vi "DriveForDistance.vi"(8 "error in (no error)":errorcluster, 9 "RobotDriveRef":T1={"RobotDriveDevRef"={"DevStatus"={"status"=FALSE, "code"=0, "source"=""}, "Motors[]"=[], "Square Inputs"=FALSE, "Max Output"=0.0}, "Control Mode"=enum."Percent VBus", "Motor Settings"={"Wheel Radius"=0.0, "Encoder Ticks Per Rev"=0.0, "Gear Ratio"=0.0, "ClimbRev"=0.0}, "Default Control Mode"=enum."Unchanged / Invalid"}, 10 "SubSystem Data":T10, 11 "Command Loop Data":cluster{"Start Time (ms)":u32, "Iterations":i32}) -> (0 "error out":errorcluster, 1 "RobotDriveRef Out":T1={"RobotDriveDevRef"={"DevStatus"={"status"=FALSE, "code"=0, "source"=""}, "Motors[]"=[], "Square Inputs"=FALSE, "Max Output"=0.0}, "Control Mode"=enum."Percent VBus", "Motor Settings"={"Wheel Radius"=0.0, "Encoder Ticks Per Rev"=0.0, "Gear Ratio"=0.0, "ClimbRev"=0.0}, "Default Control Mode"=enum."Unchanged / Invalid"}, 2 "Wait Time":dbl, 3 "Finished":bool, 5 "Left Setpoint":dbl)   [LabVIEW 2015]
uses:
  Drive Setpoints.ctl
  Drive Operations.ctl
  Advanced Drive VIs/RobotDrive Type Def.ctl
  <vilib>/Rock Robotics/WPI/MotorControl/WPI_MotorControlDeviceRef.ctl
  <vilib>/Rock Robotics/WPI/MotorControl/WPI_MotorControlType.ctl
  <vilib>/Rock Robotics/SystemInterfaces/DIO/FPGA_DIOPWMChannel.ctl
  <vilib>/Rock Robotics/WPI/PWM/WPI_PWMDeadband.ctl
  <vilib>/Rock Robotics/WPI/CAN/Jaguar/SubVIs/WPI_CANJaguar_ControlMode.ctl
  <vilib>/Rock Robotics/WPI/CAN/TalonSRX/WPI_CANTalonSRX_APIControlMode.ctl
  Advanced Drive VIs/Drive Motor Settings.ctl
panel:
  out "x*y":dbl
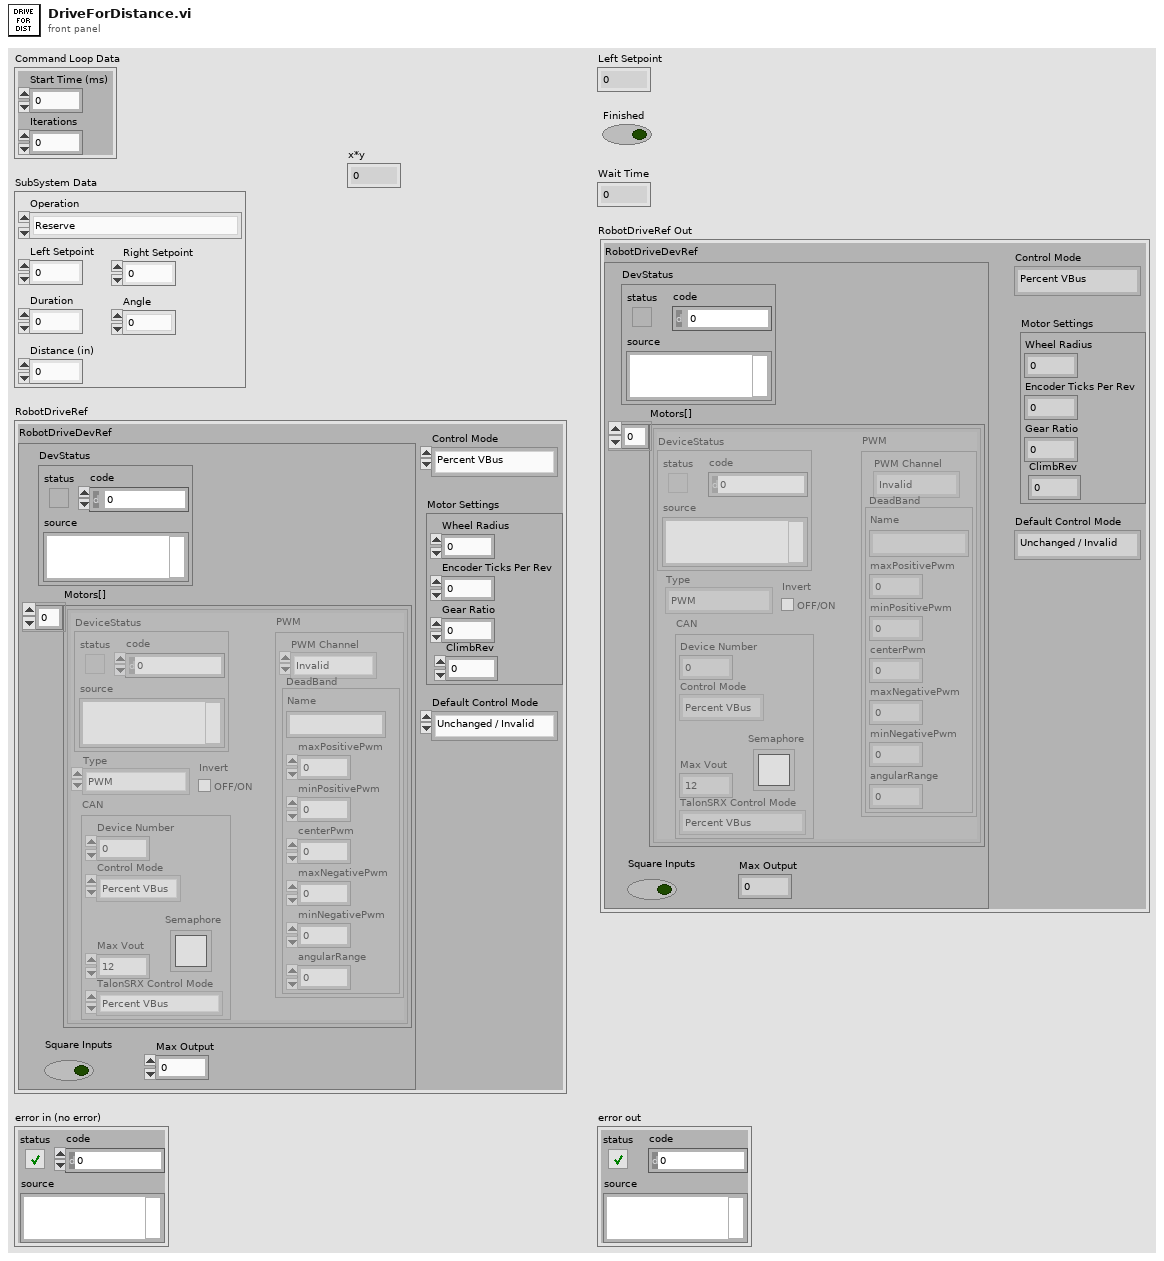
[diagram p1: front panel]
types:
  T1 = typedef "RobotDrive Type Def.ctl" = cluster{"RobotDriveDevRef":cluster{"DevStatus":errorcluster, "Motors[]":T2[], "Square Inputs":bool, "Max Output":dbl}, "Control Mode":T8, "Motor Settings":T9, "Default Control Mode":T8}
  T2 = typedef "WPI_MotorControlDeviceRef.ctl" = cluster{"DeviceStatus":errorcluster, "Type":T3, "PWM":cluster{"PWM Channel":T4, "DeadBand":T5}, "CAN":cluster{"Device Number":u8, "Control Mode":T6, "Semaphore":T7, "Max Vout":dbl, "TalonSRX Control Mode":T8}, "Invert":bool}
  T3 = typedef "WPI_MotorControlType.ctl" = enum16{"PWM", "CAN", "CANTalonSRX"}
  T4 = typedef "FPGA_DIOPWMChannel.ctl" = enum8{"PWM 0", "PWM 1", "PWM 2", "PWM 3", "PWM 4", "PWM 5", "PWM 6", "PWM 7", "PWM 8", "PWM 9", "PWM MXP 0", "PWM MXP 1", "PWM MXP 2", "PWM MXP 3", "PWM MXP 4", "PWM MXP 5", "PWM MXP 6", "PWM MXP 7", "PWM MXP 8", "PWM MXP 9", "Invalid"}
  T5 = typedef "WPI_PWMDeadband.ctl" = cluster{"Name":string, "maxPositivePwm":i32, "minPositivePwm":i32, "centerPwm":i32, "maxNegativePwm":i32, "minNegativePwm":i32, "angularRange":u16}
  T6 = typedef "WPI_CANJaguar_ControlMode.ctl" = enum8{"Percent VBus", "Current", "Speed", "Position", "Voltage"}
  T7 = typedef "Semaphore RefNum" = refnum<k1>
  T8 = typedef "WPI_CANTalonSRX_APIControlMode.ctl" = enum8{"Percent VBus", "Speed", "Position", "Slave", "Unchanged / Invalid", "Voltage Compensation", "Current", "Motion Profile"}
  T9 = typedef "Drive Motor Settings.ctl" = cluster{"Wheel Radius":dbl, "Encoder Ticks Per Rev":dbl, "Gear Ratio":dbl, "ClimbRev":dbl}
  T10 = typedef "Drive Setpoints.ctl" = cluster{"Operation":T11, "Left Setpoint":dbl, "Right Setpoint":dbl, "Duration":dbl, "Angle":dbl, "Distance (in)":dbl}
  T11 = typedef "Drive Operations.ctl" = enum16{"Reserve", "Read Current", "Immediate", "Drive for Time", "Drive for Distance", "Turn Degrees"}
  T12 = typedef "WPI_CANTalonSRX_GlobalStatus.ctl" = cluster{"Applied Throttle":dbl, "Module Enabled":bool, "CAN Error":errorcluster, "Closed Loop Error":dbl, "Forward Limit Switch Closed":bool, "Reverse Limit Switch Closed":bool, "Sensor Position":dbl, "Sensor Velocity":dbl, "Current":dbl, "Sticky Fault - Over Temp":bool, "Sticky Fault - Under Voltage":bool, "Sticky Fault - Forward Limit":bool, "Sticky Fault - Reverse Limit":bool, "Sticky Fault - Forward Soft Limit":bool, "Sticky Fault - Reverse Soft Limit":bool, "Brake is Enabled":bool, "Encoder Position":dbl, "Encoder Velocity":dbl, "Encoder Index Count":dbl, "Encoder A Pin State":bool, "Encoder B Pin State":bool, "Encoder Index Pin State":bool, "Analog In":dbl, "Analog In Velocity":dbl, "Temperature (C)":dbl, "Battery Voltage":dbl, "Control 5 Is Supported":bool, "Current Profile Slot Select":dbl, "Pos Div 8":bool, "Vel Div 4":bool, "Pulse Width Position":i32, "Pulse Width Velocity":i32, "Pulse Width Rise To Rise (us)":i32, "Pulse Width Rise To Fall (us)":i32, "Mot Prof Active Is Under Run":bool, "Mot Prof Active Has Under Run":bool, "Mot Prof Active Is Last":bool, "Mot Prof Active Velocity Only":bool, "Mot Prof Active Is Valid":bool, "Mot Prof Buffer Is Full":bool, "Mot Prof Active Profile Slot Select":i32, "Mot Prof NextID":i32, "Mot Prof Count":i32, "Mot Prof Active Velocity":dbl, "Mot Prof Active Position":dbl, "Mot Prof Output Enable":i32}
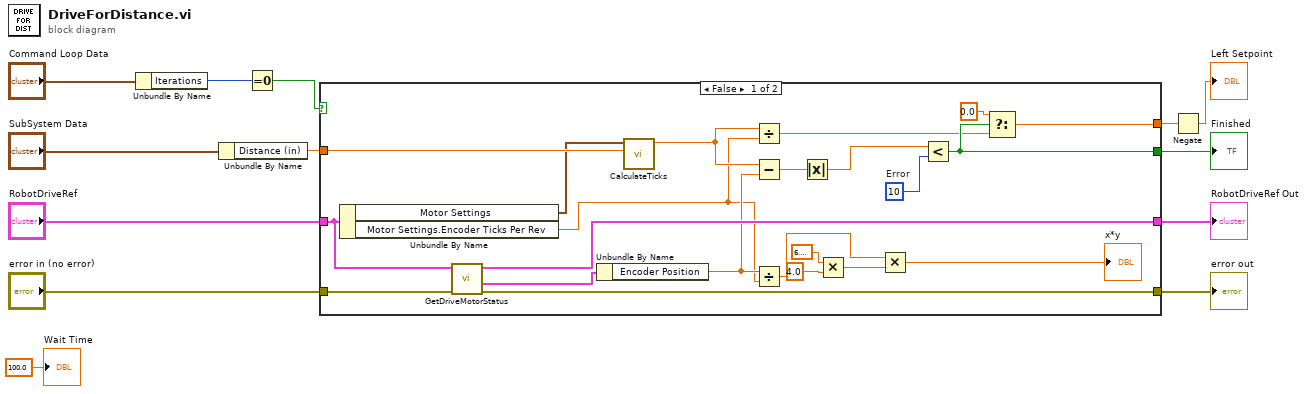
[diagram p0: block diagram]
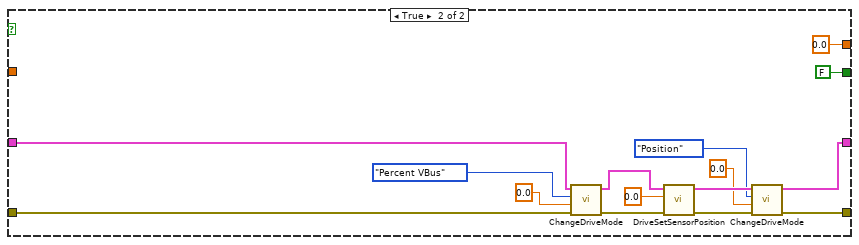
[diagram p2: hidden frame]
diagram:
  n1 = Unbundle By Name("Command Loop Data") -> ("Iterations"=w7:i32)
  n2 = Unbundle By Name("SubSystem Data") -> ("Distance (in)"=w13:dbl)
  n3 = Equal To 0?(x=w7) -> (x = 0?=w6:bool)
  n4 = case shown="False" w6 {
    tunnel: w13 -> [w31 _]
    tunnel: [w34 FALSE ("ignore previous (F)")] -> w4
    tunnel: [w32 0.0 ("Left Setpoint")] -> w2
    tunnel: "RobotDriveRef" -> [w28 w41]
    tunnel: [w29 w44] -> w9
    tunnel: "error in (no error)" -> [w27 w39]
    tunnel: [w26 w42] -> w11
    frame False {
      w35 = 10  # Error
      n5 = Unbundle By Name(w28) -> ("Motor Settings"=w25:T9, "Motor Settings.Encoder Ticks Per Rev"=w19:dbl)
      n6 = call "GetDriveMotorStatus.vi"("error in (no error)"=w27, "RobotDriveRef In"=w28) -> ("error out"=w26:errorcluster, "Right"=w21:T12, "RobotDriveRef Out"=w29:T1)  [unwired: 6 in, 1 out]
      n7 = Unbundle By Name(w21) -> ("Encoder Position"=w20:dbl)
      n8 = call "CalculateTicks.vi"("Distance (in)"=w31, "Motor Settings"=w25) -> ("Ticks"=w22:dbl)  [unwired: 9 in]
      n9 = Divide(x=w22, y=w19) -> (x/y=w30:dbl)
      n10 = Subtract(x=w22, y=w20) -> (x-y=w23:dbl)
      n11 = Divide(x=w20, y=w19) -> (x/y=w18:dbl)
      n12 = Absolute Value(x=w23) -> (abs(x)=w24:dbl)
      n13 = Multiply(x=6.283185307179586, y=4.0) -> (x*y=w15:dbl)
      n14 = Multiply(x=w18, y=w15) -> (x*y=→"x*y":dbl)
      n15 = Less?(x=w24, y=w35) -> (x < y?=w34:bool)
      n16 = Select(t=0.0, s=w34, f=w30) -> (s? t:f=w32:dbl)
    }
    frame True {
      n17 = call "ChangeDriveMode.vi"("error in (no error)"=w39, "Output"=0.0, "Control Mode"=WPI_CANTalonSRX_APIControlMode."Percent VBus", "RobotDriveRef"=w41) -> ("error out"=w38:errorcluster, "RobotDriveRef Out"=w40:T1)  [unwired: 6 in]
      n18 = call "DriveSetSensorPosition.vi"("error in (no error)"=w38, "New Sensor Position"=0.0, "RobotDriveRef In"=w40) -> ("error out"=w43:errorcluster, "RobotDriveRef Out"=w47:T1)  [unwired: 7 in]
      n19 = call "ChangeDriveMode.vi"("error in (no error)"=w43, "Output"=0.0, "Control Mode"=WPI_CANTalonSRX_APIControlMode."Position", "RobotDriveRef"=w47) -> ("error out"=w42:errorcluster, "RobotDriveRef Out"=w44:T1)  [unwired: 6 in]
    }
  }
  "error out" <- w11
  "RobotDriveRef Out" <- w9
  "Finished" <- w4
  n20 = Negate(x=w2) -> (-x=→"Left Setpoint":dbl)
  "Wait Time" <- 100.0
